vi "GMaps API Open.vi"(5 "error in (no error)":errorcluster) -> (14 "GMaps API out":refnum<class "GMaps API.lvclass">, 19 "error out":errorcluster)   [LabVIEW 2016, in "GMaps API.lvclass"]
doc: "Initializes the Google Maps API parameters to their default values."
uses:
  GMaps API.lvclass
  GMaps API.lvclass/GMaps API.ctl
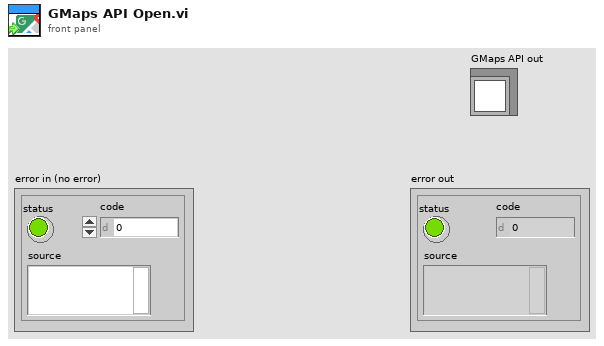
[diagram p1: front panel]
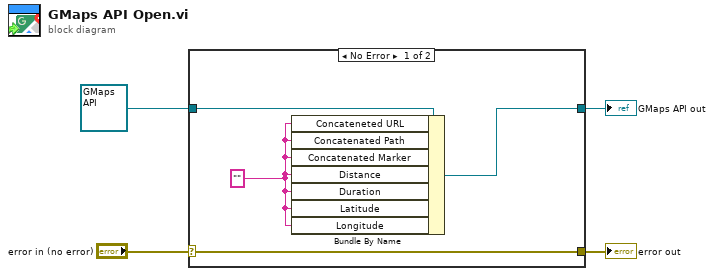
[diagram p0: block diagram]
diagram:
  n1 = case shown="No Error" "error in (no error)" {
    selector: "error in (no error)" -> [w8 w10]
    tunnel: [w8 w10] -> w3
    tunnel: [w5 w9] -> w1
    tunnel: refnum<class "GMaps API.lvclass"> refnum ("GMaps API in") -> [w7 w9]
    frame No Error {
      w6 = ""
      n2 = Bundle By Name(cluster=w7, "Concateneted URL"=w6, "Concatenated Path"=w6, "Concatenated Marker"=w6, "Distance"=w6, "Duration"=w6, "Latitude"=w6, "Longitude"=w6) -> (w5:refnum<class "GMaps API.lvclass">)
    }
    frame Error {
    }
  }
  "error out" <- w3
  "GMaps API out" <- w1
